vi "Find Item Locations by Path.vi"(5 "Insertion point if not found":bool, 6 "Only return first found":bool, 7 "Path":string, 8 "error in (no error)":errorcluster, 10 "Object Offset":i32, 11 "JSON":string) -> (0 "error out":errorcluster, 1 "Items":T1[](array[typedef]))   [LabVIEW 2017, in "JSONtext.lvlib"]
uses:
  JSONtext.lvlib
  Found Items.ctl
  Parsing State.ctl
  support/Trim Whitespace__JSONtext.vi
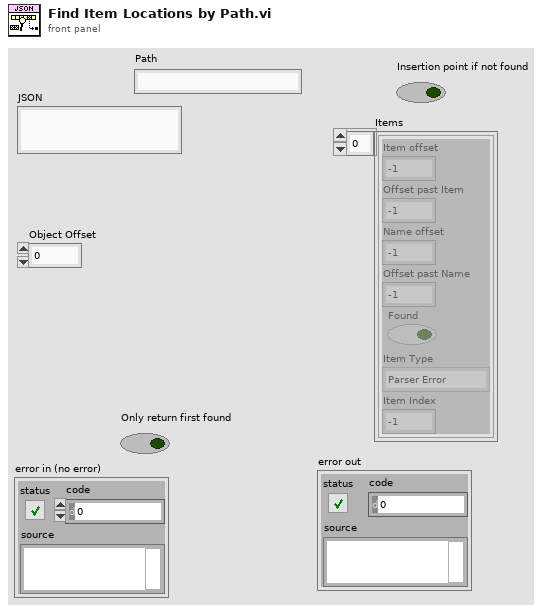
[diagram p1: front panel]
types:
  T1 = typedef "JSONtext.lvlib/Found Items.ctl" = cluster{"Item offset":i32, "Offset past Item":i32, "Name offset":i32, "Offset past Name":i32, "Found":bool, "Item Type":T2, "Item Index":i32}
  T2 = typedef "JSONtext.lvlib/Parsing State.ctl" = enum16{"Parser Error", "Object", "Array", "String", "Number/Other", "Leading Whitespace", "Object end", "Array end", "Value end"}
  T3 = cluster{"Type":T2, "Value start":i32, "Offset":i32}[]
  T4 = cluster{"Type":T2, "Value start":i32, "Offset":i32}
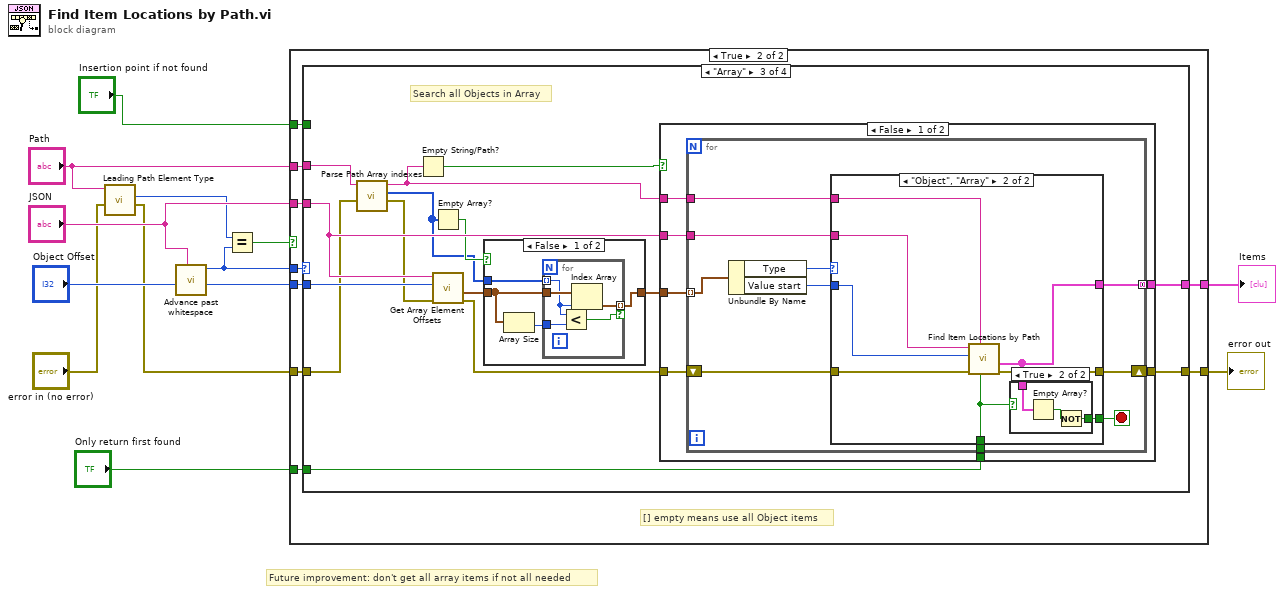
[diagram p0: block diagram]
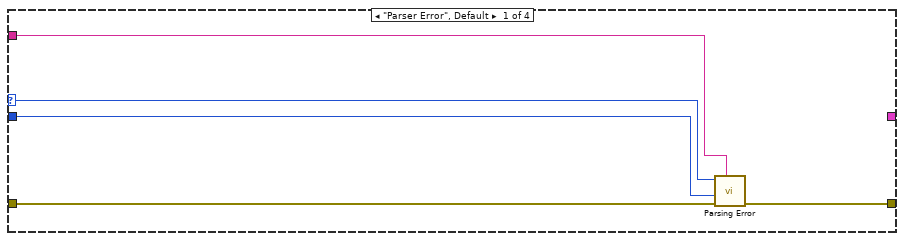
[diagram p3: hidden frame]
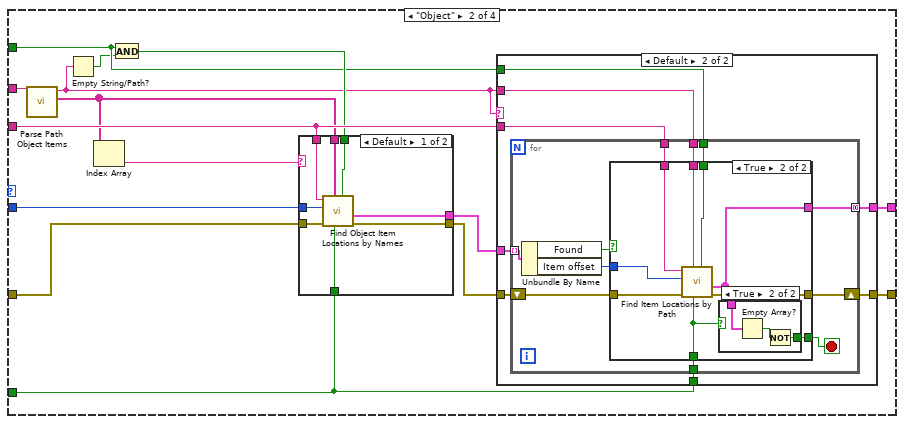
[diagram p4: hidden frame]
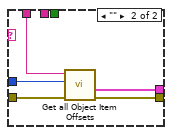
[diagram p5: hidden frame]
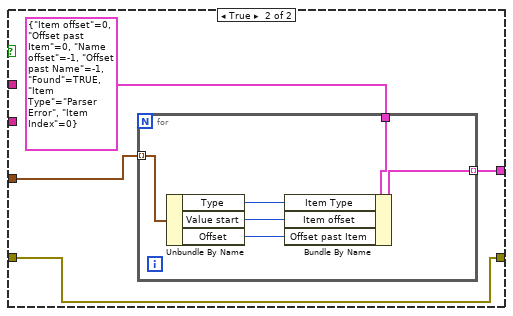
[diagram p12: hidden frame]
diagram:
  # "Future improvement: don't get all array items if not all needed"
  n1 = call "Leading Path Element Type.vi"("error in (no error)"="error in (no error)", "Path"="Path") -> ("error out"=w4:errorcluster, "Path Element Type"=w2:T2)  [unwired: 8 in]
  n2 = call "Advance past whitespace.vi"("JSON"="JSON", "Offset"="Object Offset") -> ("Offset of first non-whitespace"=w10:i32, "Parser State"=w3:T2)  [unwired: 8 in]
  n3 = Equal?(x=w2, y=w3) -> (x = y?=w1:bool)
  n4 = case shown="True" w1 {
    tunnel: [_ w23] -> w12
    tunnel: "JSON" -> [_ w22]
    tunnel: w10 -> [_ w21]
    tunnel: [w14 w20] -> w9
    tunnel: "Only return first found" -> [_ w19]
    tunnel: "Insertion point if not found" -> [_ w18]
    tunnel: "Path" -> [_ w17]
    tunnel: w4 -> [w14 w16]
    tunnel: w3 -> [_ w15]
    frame False {
    }
    frame True {
      # "[] empty means use all Object items"
      n5 = case shown="\"Array\"" w15 {
        selector: w15 -> [w26 _ _ _]
        tunnel: [_ w42 w104 _] -> w23
        tunnel: w22 -> [w24 w41 w101 _]
        tunnel: w21 -> [w25 w38 w103 _]
        tunnel: w16 -> [w28 w40 w98 w155]
        tunnel: [w27 w43 w105 w155] -> w20
        tunnel: w17 -> [_ w39 w99 _]
        tunnel: w19 -> [_ w33 w100 _]
        tunnel: w18 -> [_ w31 _ _]
        frame "Parser Error", Default {
          n6 = call "Parsing Error.vi"("JSON"=w24, "error in (no error)"=w28, "Offset past match"=w25, "State"=w26) -> ("error out"=w27:errorcluster)  [unwired: 7 in]
        }
        frame "Object" {
          n7 = call "Parse Path Object Items.vi"("Path with leading Object element"=w39) -> ("<JSON>items names"=w35:string[], "Rest or Path"=w29:string)  [unwired: 8 in, 1 out]
          n8 = Empty String/Path?(string/path=w29) -> (empty?=w30:bool)
          n9 = Index Array(array=w35) -> (element=w34:string)  [unwired: 1 in]
          n10 = And(x=w31, y=w30) -> (x .and. y?=w32:bool)
          n11 = case shown="Default" w34 {
            tunnel: w41 -> [w51 w56]
            tunnel: w40 -> [w50 w54]
            tunnel: w38 -> [w49 w55]
            tunnel: w35 -> [w48 _]
            tunnel: [w47 w53] -> w37
            tunnel: [w46 w52] -> w36
            tunnel: w33 -> [w45 _]
            tunnel: w32 -> [w44 _]
            frame Default {
              n12 = call "Find Object Item Locations by Names.vi"("Insertion point if not found"=w44, "Only return first found"=w45, "Item Names <JSON>"=w48, "error in (no error)"=w50, "Object Offset"=w49, "JSON"=w51) -> ("error out"=w47:errorcluster, "Items"=w46:T1[])  [unwired: 4 in]
            }
            frame "" {
              n13 = call "Get all Object Item Offsets.vi"("error in (no error)"=w54, "Offset"=w55, "JSON"=w56) -> ("error out"=w53:errorcluster, "Items"=w52:T1[])  [unwired: 6 in, 1 out]
            }
          }
          n14 = case shown="Default" w29 {
            tunnel: [w57 w66] -> w43
            tunnel: [w58 w65] -> w42
            tunnel: w41 -> [_ w64]
            tunnel: w29 -> [_ w63]
            tunnel: w37 -> [w57 w62]
            tunnel: w36 -> [w58 w61]
            tunnel: w33 -> [_ w60]
            tunnel: w31 -> [_ w59]
            frame "" {
            }
            frame Default {
              n15 = for {
                tunnel: [w76] -> w65 mode=concatenating
                tunnel: w64 -> [w75]
                tunnel: w63 -> [w74]
                tunnel: w61 -> [w72] mode=indexing
                shift-right: [w77] -> w66
                shift-left: w62 -> [w73]
                tunnel: w60 -> [w69]
                tunnel: w59 -> [w67]
                stop <- w68 stop-if-true
                n16 = Unbundle By Name(w72) -> ("Found"=w71:bool, "Item offset"=w70:i32)
                n17 = case shown="True" w71 {
                  tunnel: [w78 w87] -> w77
                  tunnel: [_ w81] -> w76
                  tunnel: w75 -> [_ w86]
                  tunnel: w74 -> [_ w85]
                  tunnel: w73 -> [w78 w84]
                  tunnel: w70 -> [_ w83]
                  tunnel: w69 -> [_ w82]
                  tunnel: [_ w80] -> w68
                  tunnel: w67 -> [_ w79]
                  frame False {
                  }
                  frame True {
                    n18 = call "Find Item Locations by Path.vi"("Insertion point if not found"=w79, "Only return first found"=w82, "Path"=w85, "error in (no error)"=w84, "Object Offset"=w83, "JSON"=w86) -> ("error out"=w87:errorcluster, "Items"=w81:T1[])  [unwired: 4 in]
                    n19 = case shown="True" w82 {
                      tunnel: w81 -> [_ w90]
                      tunnel: [_ w88] -> w80
                      frame False {
                      }
                      frame True {
                        n20 = Empty Array?(array=w90) -> (empty?=w89:bool)
                        n21 = Not(x=w89) -> (.not. x?=w88:bool)
                      }
                    }
                  }
                }
              }
            }
          }
        }
        frame "Array" {
          # "Search all Objects in Array"
          n22 = call "Parse Path Array indexes.vi"("error in (no error)"=w98, "Path with leading Array element"=w99) -> ("error out"=w97:errorcluster, "Indexes (empty means use all)"=w91:i32[], "Rest or Path"=w96:string)  [unwired: 7 in]
          n23 = Empty String/Path?(string/path=w96) -> (empty?=w95:bool)
          n24 = Empty Array?(array=w91) -> (empty?=w94:bool)
          n25 = call "Get Array Element Offsets.vi"("error in (no error)"=w97, "Offset"=w103, "JSON"=w101) -> ("error out"=w102:errorcluster, "Elements"=w92:T3)  [unwired: 6 in, 1 out]
          n26 = case shown="False" w94 {
            tunnel: [w108 w115] -> w93
            tunnel: w92 -> [w107 w115]
            tunnel: w91 -> [w109 _]
            frame False {
              n27 = Array Size(array=w107) -> (size(s)=w106:i32)
              n28 = for {
                tunnel: w109 -> [w112] mode=indexing
                tunnel: w107 -> [w114]
                tunnel: [w113] -> w108 mode=indexing if=w110
                tunnel: w106 -> [w111]
                n29 = Less?(x=w112, y=w111) -> (x < y?=w110:bool)
                n30 = Index Array(array=w114, index=w112) -> (element=w113:T4)
              }
            }
            frame True {
              # "No indexes means\nuse all"
            }
          }
          n31 = case shown="False" w95 {
            tunnel: [w122 w145] -> w105
            tunnel: [w121 w146] -> w104
            tunnel: w93 -> [w120 w148]
            tunnel: w102 -> [w119 w145]
            tunnel: w101 -> [w118 _]
            tunnel: w100 -> [w117 _]
            tunnel: w96 -> [w116 _]
            frame False {
              n32 = for {
                tunnel: [w130] -> w121 mode=concatenating
                shift-right: [w131] -> w122
                shift-left: w119 -> [w132]
                tunnel: w116 -> [w129]
                tunnel: w120 -> [w128] mode=indexing
                tunnel: w118 -> [w126]
                tunnel: w117 -> [w124]
                stop <- w123 stop-if-true
                n33 = Unbundle By Name(w128) -> ("Type"=w127:T2, "Value start"=w125:i32)
                n34 = case shown="\"Object\", \"Array\"" w127 {
                  tunnel: w132 -> [w133 w141]
                  tunnel: [w133 w140] -> w131
                  tunnel: [_ w136] -> w130
                  tunnel: w129 -> [_ w139]
                  tunnel: w126 -> [_ w138]
                  tunnel: w125 -> [_ w137]
                  tunnel: w124 -> [_ w134]
                  tunnel: [_ w135] -> w123
                  frame "Parser Error", Default {
                  }
                  frame "Object", "Array" {
                    n35 = call "Find Item Locations by Path.vi"("Only return first found"=w134, "Path"=w139, "error in (no error)"=w141, "Object Offset"=w137, "JSON"=w138) -> ("error out"=w140:errorcluster, "Items"=w136:T1[])  [unwired: 5 in]
                    n36 = case shown="True" w134 {
                      tunnel: w136 -> [_ w144]
                      tunnel: [_ w142] -> w135
                      frame False {
                      }
                      frame True {
                        n37 = Empty Array?(array=w144) -> (empty?=w143:bool)
                        n38 = Not(x=w143) -> (.not. x?=w142:bool)
                      }
                    }
                  }
                }
              }
            }
            frame True {
              n39 = for {
                tunnel: w148 -> [w154] mode=indexing
                tunnel: T1 {"Item offset"=0, "Offset past Item"=0, "Name offset"=-1, "Offset past Name"=-1, "Found"=TRUE, "Item Type"=enum."Parser Error", "Item Index"=0} -> [w153]
                tunnel: [w152] -> w146 mode=indexing
                n40 = Unbundle By Name(w154) -> ("Type"=w149:T2, "Value start"=w150:i32, "Offset"=w151:i32)
                n41 = Bundle By Name(cluster=w153, "Item Type"=w149, "Item offset"=w150, "Offset past Item"=w151) -> (w152:T1)
              }
            }
          }
        }
        frame "String", "Number/Other" {
          # "Not an object or Array so Path ends here\n\n--> throw error?"
        }
      }
    }
  }
  "Items" <- w12
  "error out" <- w9
